vi "Read Coils.vi"(8 "error in":errorcluster, 9 "number of inputs":u16, 10 "starting address":u16, 11 "Modbus master in":refnum<class "Modbus Master.lvclass">) -> (0 "error out":errorcluster, 2 "coils":bool[](array[boolean]), 3 "Modbus master out":refnum<class "Modbus Master.lvclass">)   [LabVIEW 2014, in "MyLib.lvlib" / "Modbus Master.lvclass"]
doc: "Reads <B>number of inputs</B> coils starting at <B>starting address</B> from the device."
uses:
  Modbus Master.lvclass
  Modbus Master.lvclass/Modbus Master.ctl
  Modbus API.lvclass/Modbus API.ctl
  Transmission Data Unit/Transmission Data Unit.lvclass
  Modbus API.lvclass
  Master Function Definition/Master Function Definition.lvclass
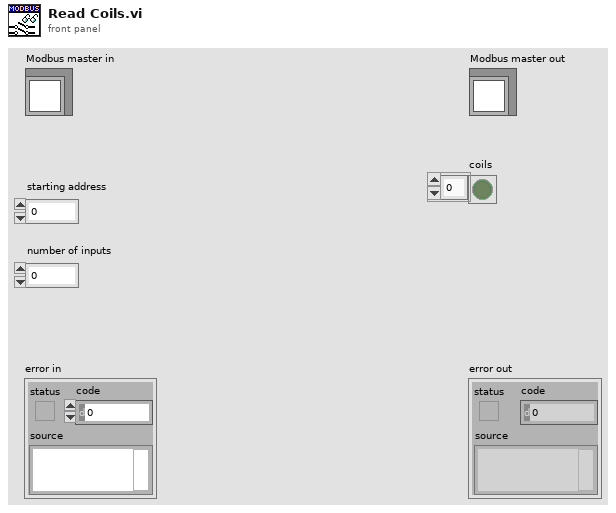
[diagram p1: front panel]
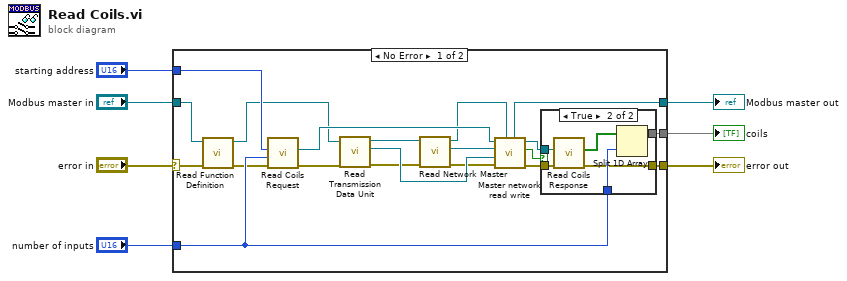
[diagram p0: block diagram]
diagram:
  n1 = case shown="No Error" "error in" {
    selector: "error in" -> [w20 w36]
    tunnel: [w19 w36] -> w5
    tunnel: [w16 w35] -> w6
    tunnel: "Modbus master in" -> [w21 w35]
    tunnel: "starting address" -> [w27 _]
    tunnel: "number of inputs" -> [w26 _]
    tunnel: [w25 _] -> w4
    frame No Error {
      n2 = call "Read Function Definition.vi"("error in"=w20, "Modbus master in"=w21) -> ("error out"=w15:errorcluster, "Modbus master out"=w11:refnum<class "Modbus Master.lvclass">)  [unwired: 7 in, 1 out]
      n3 = call "Read Coils Request.vi"("error in"=w15, "Number of coils"=w26, "Starting Address"=w27) -> ("error out"=w9:errorcluster, "modbus data unit out"=w24:refnum<class "Modbus Data Unit.lvclass">)  [unwired: 7 in]
      n4 = call "Read Transmission Data Unit.vi"("error in"=w9, "Modbus instance in"=w11) -> ("error out"=w13:errorcluster, "transmission data unit"=w18:refnum<class "Transmission Data Unit.lvclass">, "Modbus instance out"=w12:refnum<class "Modbus Master.lvclass">)  [unwired: 7 in]
      n5 = call "Read Network Master.vi"("error in"=w13, "Modbus master in"=w12) -> ("error out"=w14:errorcluster, "network master"=w17:refnum<class "Network Master.lvclass">, "Modbus master out"=w10:refnum<class "Modbus Master.lvclass">)  [unwired: 7 in]
      n6 = call "Master network read write.vi"("Modbus master in"=w10, "error in"=w14, "transmission data unit in"=w18, "network master in"=w17, "Modbus data unit in"=w24) -> ("error out"=w22:errorcluster, "PDU Valid?"=w8:bool, "Modbus data unit out"=w23:refnum<class "Modbus Data Unit.lvclass">, "Modbus master out"=w16:refnum<class "Modbus Master.lvclass">)  [unwired: 3 in]
      n7 = case shown="True" w8 {
        tunnel: w26 -> [_ w34]
        tunnel: [_ w33] -> w25
        tunnel: w23 -> [_ w31]
        tunnel: w22 -> [w28 w30]
        tunnel: [w28 w29] -> w19
        frame False {
        }
        frame True {
          n8 = call "Read Coils Response.vi"("error in"=w30, "modbus data unit in"=w31) -> ("error out"=w29:errorcluster, "Data"=w32:bool[])  [unwired: 8 in]
          n9 = Split 1D Array(array=w32, index=w34) -> (first subarray=w33:bool[])  [unwired: 1 out]
        }
      }
    }
    frame Error {
    }
  }
  "error out" <- w5
  "Modbus master out" <- w6
  "coils" <- w4
